vi "test.ingest_mcapProtobufTimeseries.vi"   [LabVIEW 2020]
uses:
  datasources/dataset/dataset.lvclass
  81c5314d-0c17-4e40-9591-806fc92e59be.vi
  Nominal Client/Nominal Client.lvclass
  40e2c779-94f0-4ff6-913c-6196809b7e71.vi
  Nominal Client/ingest_mcapProtobufTimeseries.vi
  datasources/source/source.lvclass
  datasources/target/target.lvclass
  nominal types/channelConfig/channelConfig.lvclass
  nominal types/channelFilter/channelFilter.lvclass
  nominal types/channelFilter/create.all.vi
  nominal types/channelFilter/create.include_id.vi
  nominal types/channelFilter/create.exclude_task.vi
  nominal types/channelFilter/create.exclude_id.vi
  nominal types/channelFilter/create.include_task.vi
  datasources/source/create_gcs.vi
  datasources/target/create_new.vi
  datasources/target/create_from_existing.vi
  datasources/source/create_s3.vi
  nominal types/properties/properties.lvclass
  nominal types/all/all.lvclass
  C:/code/labview-client/lv_src/nominal types/channelFilter/channelFilter.lvclass
  C:/code/labview-client/lv_src/Nominal Client/datasources/payload/payload.lvclass
  C:/code/labview-client/lv_src/nominal types/all/all.lvclass
  nominal types/include/include.lvclass
  C:/code/labview-client/lv_src/nominal types/include/include.lvclass
  nominal types/exclude/exclude.lvclass
  C:/code/labview-client/lv_src/nominal types/exclude/exclude.lvclass
  datasources/s3/s3.lvclass
  C:/code/labview-client/lv_src/Nominal Client/datasources/source/source.lvclass
  C:/code/labview-client/lv_src/Nominal Client/datasources/s3/s3.lvclass
  datasources/gcs/gcs.lvclass
  C:/code/labview-client/lv_src/Nominal Client/datasources/gcs/gcs.lvclass
types:
  T1 = cluster{"dataset":refnum<class "dataset.lvclass">, "channelConfig":refnum<class "channelConfig.lvclass">}
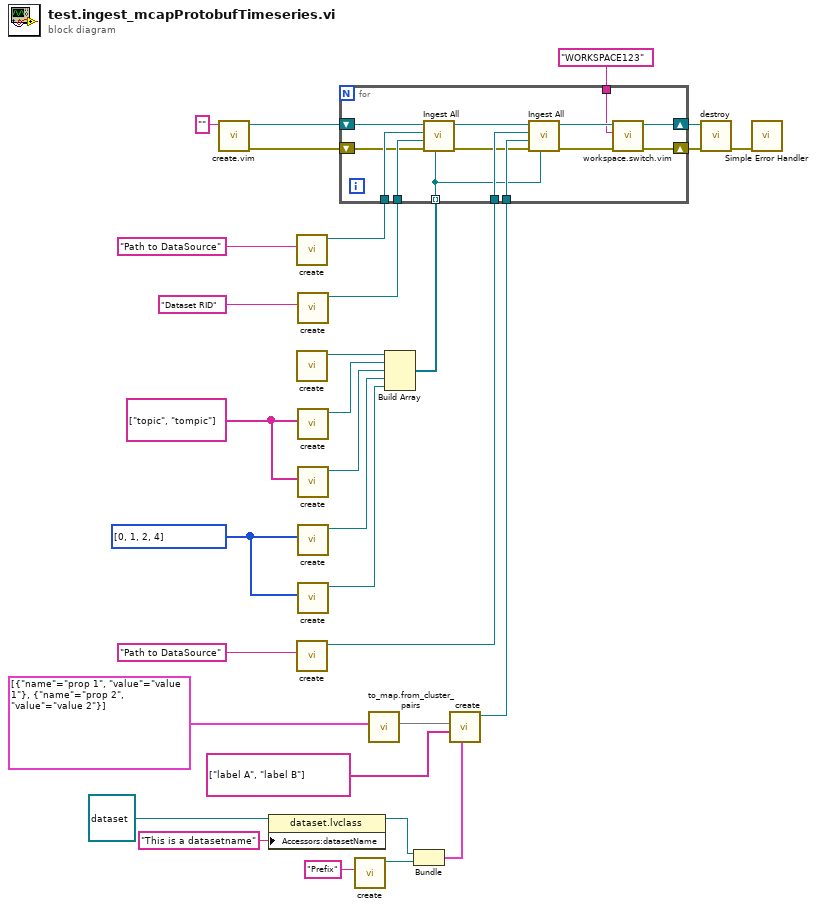
[diagram p0: block diagram]
diagram:
  w4 = i32[] [0, 1, 2, 4] ("IDs")
  w5 = string[] ["topic", "tompic"] ("topic")
  n1 = call "create.vim"("API Token (string or path)"="") -> ("error out"=w27:errorcluster, "Nominal Client"=w28:refnum<class "Nominal Client.lvclass">)  [unwired: 9 in]
  n2 = property class="dataset.lvclass"(reference=refnum<class "dataset.lvclass"> refnum ("dataset"), "Accessors:datasetName"="This is a datasetname" ("datasetName")) -> (reference out=w23:refnum<class "dataset.lvclass">)  [unwired: 1 in, 1 out]
  n3 = call-poly "create.vi"("Path"="Path to DataSource") -> ("source"=w12:refnum<class "s3.lvclass">)  [unwired: 10 in]
  n4 = call-poly "create.vi"() -> ("all"=w22:refnum<class "all.lvclass">)  [unwired: 11 in]
  n5 = call-poly "create.vi"("Path"="Path to DataSource") -> ("source"=w10:refnum<class "gcs.lvclass">)  [unwired: 10 in]
  n6 = call-poly "create.vi"("dataset RID"="Dataset RID" ("RID")) -> ("Existing Target"=w14:refnum<class "target.lvclass">)  [unwired: 10 in]
  n7 = call-poly "create.vi"("topic"=w5) -> ("Include Filter"=w21:refnum<class "include.lvclass">)  [unwired: 10 in]
  n8 = call-poly "create.vi"("topic"=w5) -> ("Exclude Filter"=w20:refnum<class "exclude.lvclass">)  [unwired: 10 in]
  n9 = call-poly "create.vi"("IDs"=w4) -> ("Include Filter"=w19:refnum<class "include.lvclass">)  [unwired: 10 in]
  n10 = call-poly "create.vi"("IDs"=w4) -> ("Exclude Filter"=w18:refnum<class "exclude.lvclass">)  [unwired: 10 in]
  n11 = call "create.vi"("prefixTreeDelimiter"="Prefix") -> ("channelConfig"=w6:refnum<class "channelConfig.lvclass">)  [unwired: 10 in]
  n12 = call "to_map.from_cluster_pairs.vi"("properties (cluster pairs)"=cluster{"name":string, "value":string}[] [{"name"="prop 1", "value"="value 1"}, {"name"="prop 2", "value"="value 2"}] ("properties")) -> ("properties (map)"=w1:map{string, string})  [unwired: 10 in]
  n13 = Build Array(w22, w21, w20, w19, w18) -> (w17:refnum<class "channelFilter.lvclass">[])
  n14 = Bundle("dataset"=w23, "channelConfig"=w6) -> (w9:T1)  [unwired: 1 in]
  n15 = call-poly "create.vi"("Optional"=w9, "Labels"=string[] ["label A", "label B"] ("labels"), "Properties"=w1) -> ("New Target"=w8:refnum<class "target.lvclass">)  [unwired: 8 in]
  n16 = for {
    tunnel: w14 -> [w45]
    tunnel: w12 -> [w44]
    tunnel: w10 -> [w43]
    tunnel: w8 -> [w42]
    shift-right: [w35] -> w29
    shift-left: w27 -> [w39]
    shift-right: [w34] -> w31
    shift-left: w28 -> [w38]
    tunnel: "WORKSPACE123" ("RID") -> [w33]
    tunnel: w17 -> [w32] mode=indexing
    n17 = call-poly "Ingest All.vi"("Channel Filter"=w32, "error in"=w39, "Target"=w45, "Source"=w44, "Nominal Client in"=w38) -> ("error out"=w40:errorcluster, "Nominal Client out"=w41:refnum<class "Nominal Client.lvclass">)  [unwired: 3 in, 2 out]
    n18 = call-poly "Ingest All.vi"("Channel Filter"=w32, "error in"=w40, "Target"=w42, "Source"=w43, "Nominal Client in"=w41) -> ("error out"=w36:errorcluster, "Nominal Client out"=w37:refnum<class "Nominal Client.lvclass">)  [unwired: 3 in, 2 out]
    n19 = call "workspace.switch.vim"("error in"=w36, "Workspace RID (string or path)"=w33, "Nominal Client in"=w37) -> ("error out"=w35:errorcluster, "Nominal Client out"=w34:refnum<class "Nominal Client.lvclass">)  [unwired: 7 in]
  }
  n20 = call "destroy.vi"("error in"=w29, "Nominal Client"=w31) -> ("error out"=w16:errorcluster)  [unwired: 9 in]
  n21 = call <vilib>:"Simple Error Handler.vi"("error in (no error)"=w16) -> ()  [unwired: 4 in, 5 out]
